vi "reconCluster.vi"(7 "Array 6":bool[](array[boolean]), 8 "Variable header":string[](array[string]), 9 "Alias":string[](array[string]), 10 "Data in":string[][](array[string]), 11 "variant in":variant) -> (1 "time":u32, 3 "variant out":variant)   [LabVIEW 2013]
uses:
  IMAQ Image.ctl
  NI_Vision_Development_Module.lvlib
panel:
  out "Img str lengths":i32[](array[numeric])
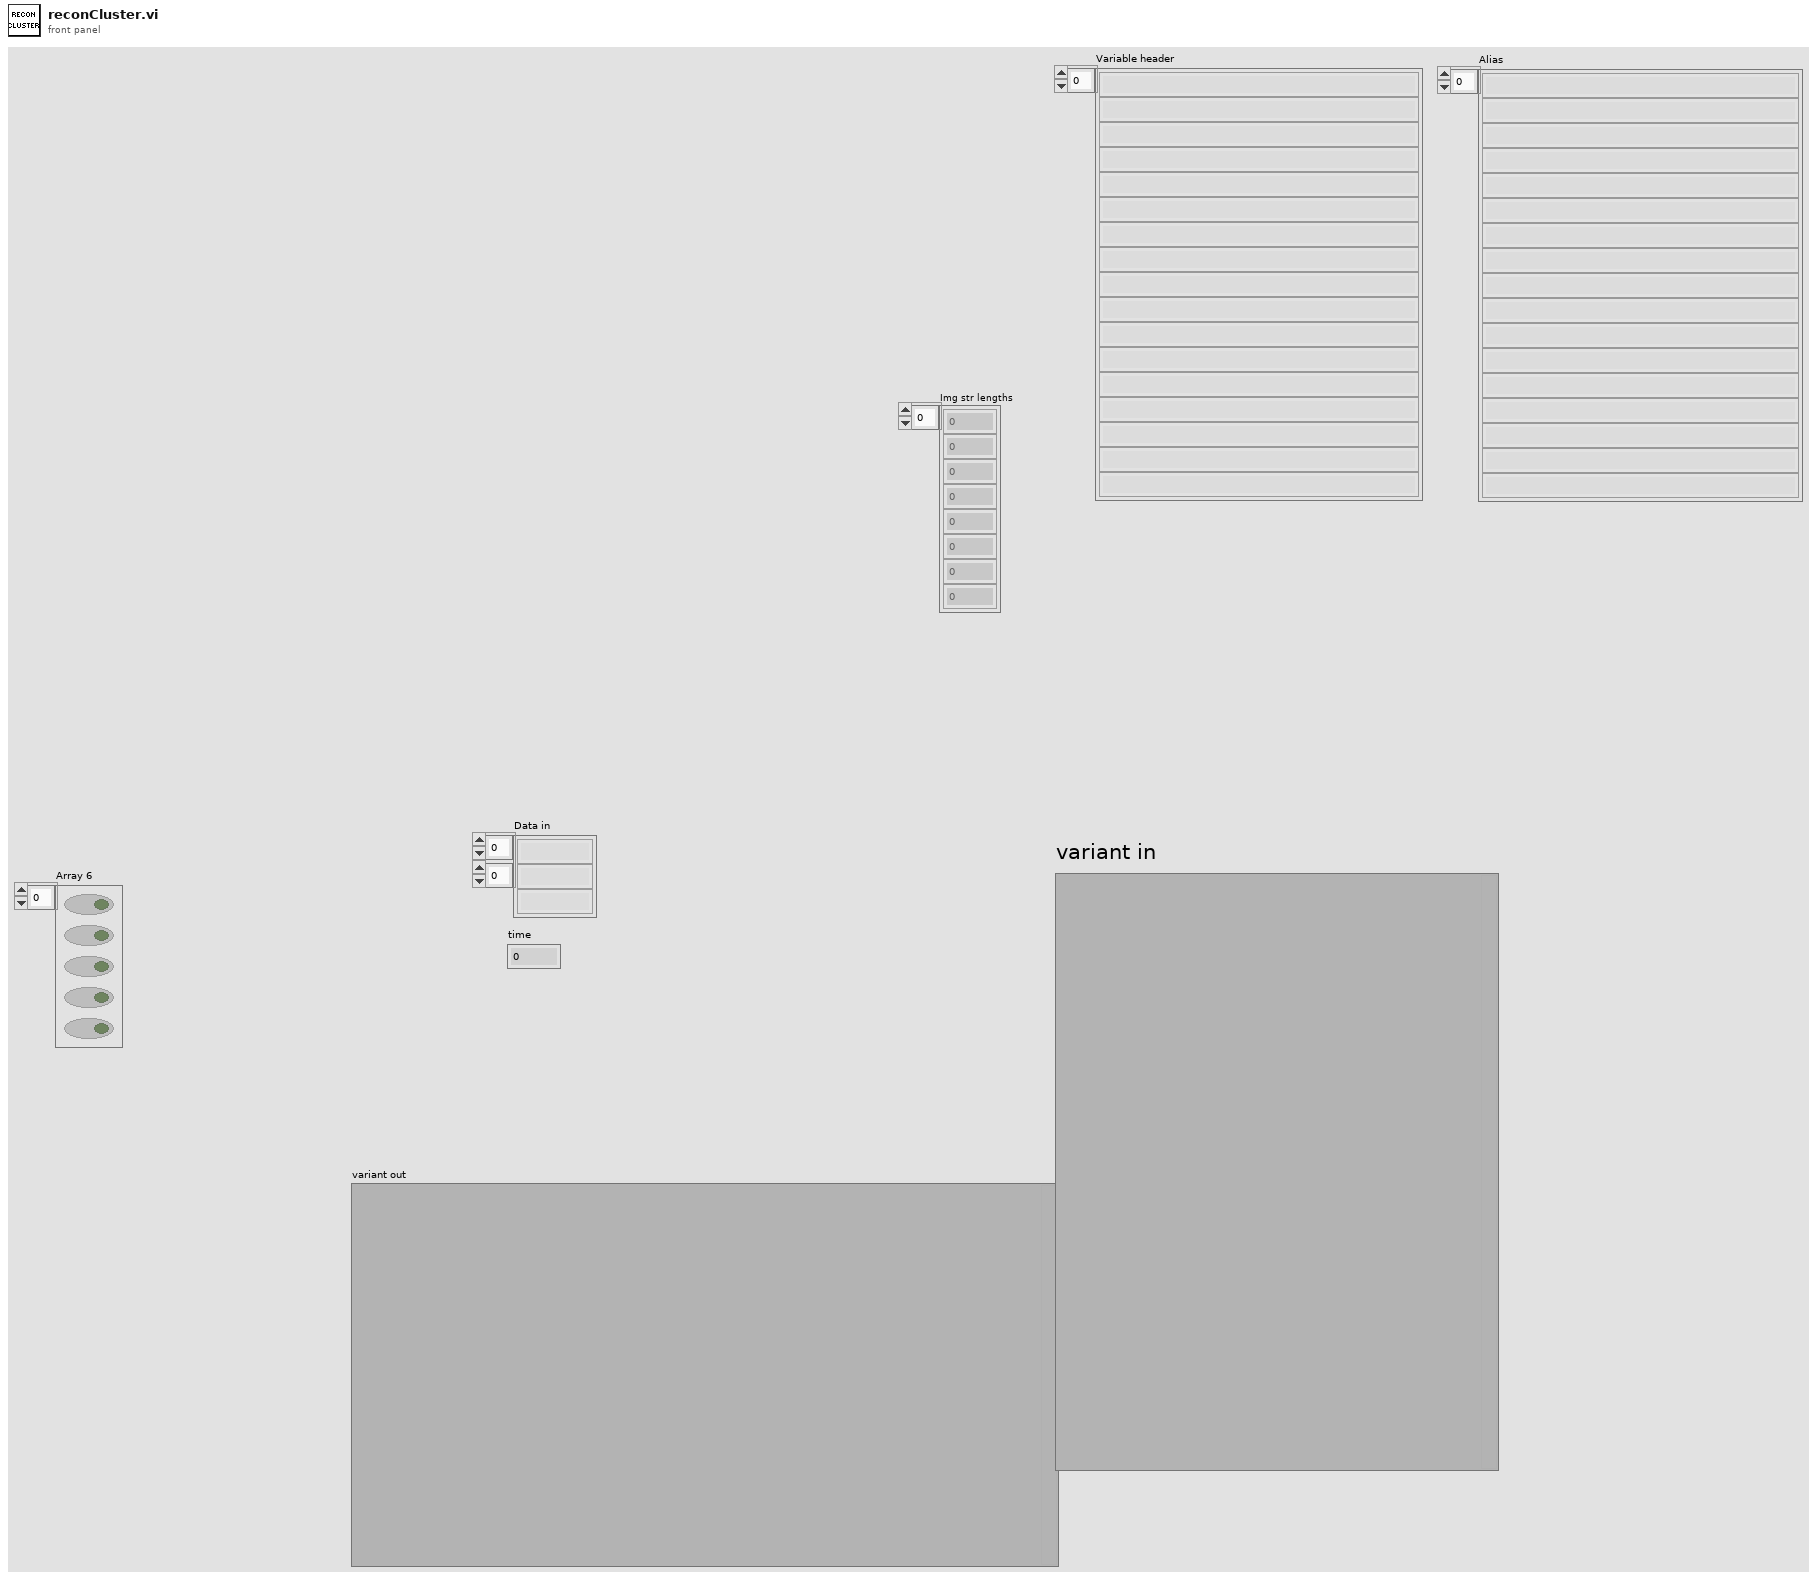
[diagram p1: front panel]
types:
  T1 = typedef "IMAQ Image.ctl" = refnum<image>
  T2 = typedef "Type Descriptor Enumeration__ogtk.ctl" = enum8{"<Null>", "I8", "I16", "I32", "I64", "U8", "U16", "U32", "U64", "SGL", "DBL", "EXT", "CSG", "CDB", "CXT", "0x0F", "0x10", "0x11", "0x12", "0x13", "0x14", "Enum U8", "Enum U16", "Enum U32", "Enum U64", "SGL PQ", "DBL PQ", "EXT PQ", "CSG PQ", "CDB PQ", "CXT PQ", "0x1F", "0x20", "Boolean", "0x22", "0x23", "0x24", "0x25", "0x26", "0x27", "0x28", "0x29", "0x2A", "0x2B", "0x2C", "0x2D", "0x2E", "0x2F", "String", "0x31", "Path", "Pict", "0x34", "0x35", "0x36", "DAQ", "0x38", "0x39", "0x3A", "0x3B", "0x3C", "0x3D", "0x3E", "0x3F", "Array", "0x41", "0x42", "0x43", "0x44", "0x45", "0x46", "0x47", "0x48", "0x49", "0x4A", "0x4B", "0x4C", "0x4D", "0x4E", "0x4F", "Cluster", "0x51", "0x52", "Variant", "Waveform", "0x55", "0x56", "0x57", "0x58", "0x59", "0x5A", "0x5B", "0x5C", "0x5D", "0x5E", "0x5F", "0x60", "0x61", "0x62", "0x63", "0x64", "0x65", "0x66", "0x67", "0x68", "0x69", "0x6A", "0x6B", "0x6C", "0x6D", "0x6E", "0x6F", "Refnum"}
  T3 = typedef "Image Type" = u32
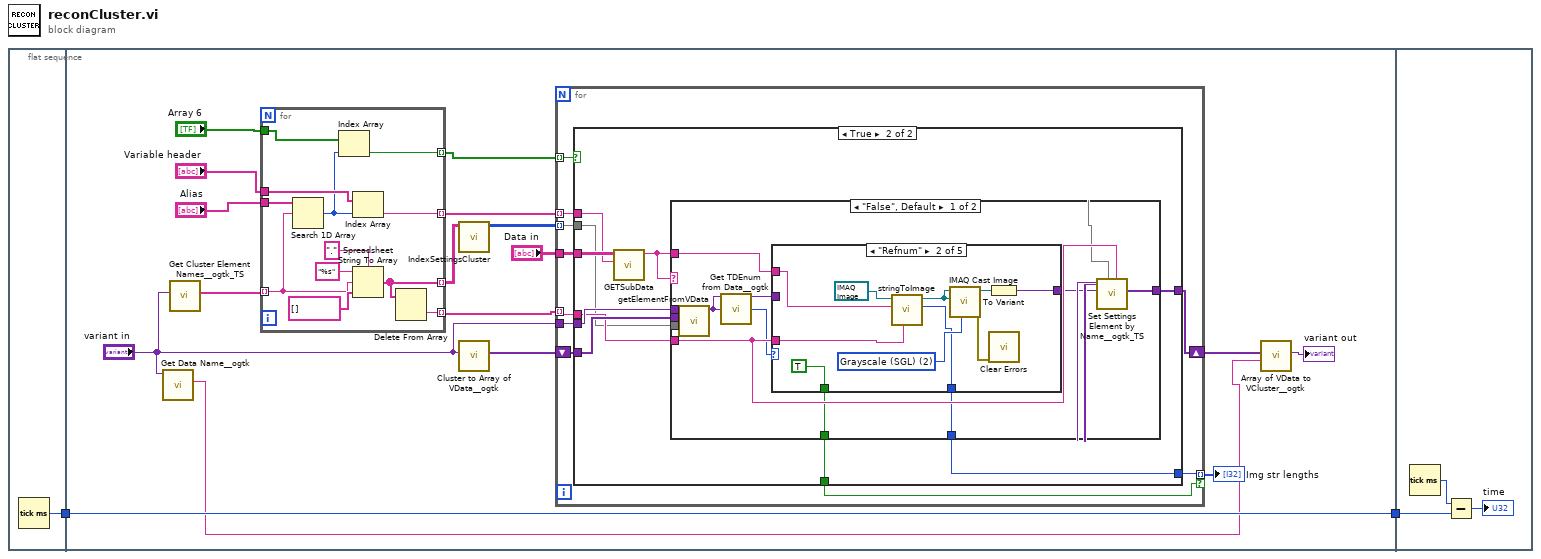
[diagram p0: block diagram]
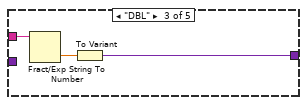
[diagram p4: hidden frame]
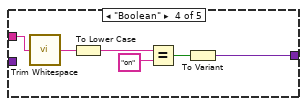
[diagram p5: hidden frame]
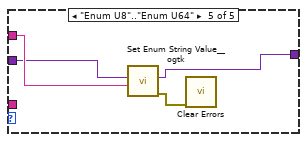
[diagram p6: hidden frame]
diagram:
  n1 = flat-sequence {
    tunnel: [w3] -> w2
    tunnel: w2 -> [w13]
    tunnel: [w13] -> w1
    tunnel: w1 -> [w90]
    frame #0 {
      n2 = Tick Count (ms)() -> (millisecond timer value=w3:u32)
    }
    frame #1 {
      n3 = call "Get Data Name__ogtk.vi"("Data"="variant in") -> ("Data Name"=w7:string)  [unwired: 8 in, 2 out]
      n4 = call "Get Cluster Element Names__ogtk_TS.vi"("Variant"="variant in") -> ("Names (Array)"=w19:string[])  [unwired: 9 in, 1 out]
      n5 = for {
        tunnel: w19 -> [w82] mode=indexing
        tunnel: [w85] -> w20 mode=indexing
        tunnel: [w84] -> w16 mode=indexing
        tunnel: "Alias" -> [w83]
        tunnel: "Variable header" -> [w81]
        tunnel: [w80] -> w9 mode=indexing
        tunnel: "Array 6" -> [w79]
        tunnel: [w77] -> w5 mode=indexing
        n6 = Search 1D Array(1D array=w83, element=w82) -> (index of element=w78:i32)  [unwired: 1 in]
        n7 = Index Array(array=w79, index=w78) -> (element=w77:bool)
        n8 = Index Array(array=w81, index=w78) -> (element=w80:string)
        n9 = Spreadsheet String To Array(delimiter (Tab)=".", format string="%s", spreadsheet string=w82, array type (2D Dbl)=string[] []) -> (array=w85:string[])
        n10 = Delete From Array(array=w85) -> (deleted portion=w84:string)  [unwired: 2 in, 1 out]
      }
      n11 = call "IndexSettingsCluster.vi"("Names Array"=w20) -> ("index Array"=w17:i32[][])  [unwired: 10 in]
      n12 = call "Cluster to Array of VData__ogtk.vi"("Cluster"="variant in") -> ("Array of VData"=w18:variant[])  [unwired: 9 in, 1 out]
      n13 = for {
        shift-right: [w30] -> w15
        shift-left: w18 -> [w28]
        tunnel: w17 -> [w27] mode=indexing
        tunnel: "variant in" -> [w29]
        tunnel: w16 -> [w24] mode=indexing
        tunnel: "Data in" -> [w26]
        tunnel: w9 -> [w25] mode=indexing
        tunnel: w5 -> [w23] mode=indexing
        tunnel: [w22] -> w4 mode=indexing if=w21
        n14 = case shown="True" w23 {
          tunnel: [w31 w41] -> w30
          tunnel: w29 -> [_ w40]
          tunnel: w28 -> [w31 w39]
          tunnel: w27 -> [_ w35]
          tunnel: w26 -> [_ w38]
          tunnel: w25 -> [_ w37]
          tunnel: w24 -> [_ w36]
          tunnel: [_ w33] -> w21
          tunnel: [_ w32] -> w22
          frame False {
          }
          frame True {
            n15 = call "GETSubData.vi"("Variable Header"=w37, "Data out"=w38) -> ("delimiter (Tab)"=w34:string)  [unwired: 9 in]
            n16 = case shown="\"False\", Default" w34 {
              tunnel: [w52 _] -> w41
              tunnel: w40 -> [w51 _]
              tunnel: w39 -> [w50 _]
              tunnel: w34 -> [w49 _]
              tunnel: w36 -> [w48 _]
              tunnel: w35 -> [w44 _]
              tunnel: [w43 _] -> w33
              tunnel: [w42 _] -> w32
              frame "False", Default {
                n17 = call "getElementFromVData.vi"("index Array 2"=w44, "Settings VData"=w50, "Cluster in"=w51) -> ("element out"=w45:variant)  [unwired: 6 in, 2 out]
                n18 = call "Get TDEnum from Data__ogtk.vi"("Data"=w45) -> ("Type Descriptor Enumeration"=w47:T2)  [unwired: 4 in]
                n19 = case shown="\"Refnum\"" w47 {
                  tunnel: w49 -> [_ w63 w66 w72 w76]
                  tunnel: w48 -> [_ w57 _ _ _]
                  tunnel: [w53 w58 w64 w67 w74] -> w46
                  tunnel: w45 -> [w53 _ _ _ w75]
                  tunnel: [_ TRUE ("element") _ _ _] -> w43
                  tunnel: [_ w54 _ _ _] -> w42
                  frame "<Null>", Default {
                  }
                  frame "Refnum" {
                    w61 = T3 2 items=["Grayscale (U8)", "Grayscale (I16)", "Grayscale (SGL)", "Complex (CSG)", "RGB (U32)", "HSL (U32)", "RGB (U64)", "Grayscale (U16)"] ("Image Type")
                    n20 = call "stringToImage.vi"("label text (image name)"=w57, "data in"=w63, "Refnum in"=T1 refnum ("Image")) -> ("length"=w54:i32, "Refnum out"=w62:T1)  [unwired: 5 in, 2 out]
                    n21 = call "IMAQ Cast Image"("Image Type"=w61, "Image Dst"=w62, "Image Src"=w62) -> ("error out"=w56:errorcluster, "Image Dst Out"=w59:T1)  [unwired: 7 in]
                    n22 = To Variant(anything=w59) -> (Variant=w58:variant)
                    n23 = call "Clear Errors.vi"("error in (no error)"=w56) -> ()  [unwired: 6 in, 1 out]
                  }
                  frame "DBL" {
                    n24 = Fract/Exp String To Number(string=w66) -> (number=w65:dbl)  [unwired: 3 in, 1 out]
                    n25 = To Variant(anything=w65) -> (Variant=w64:variant)
                  }
                  frame "Boolean" {
                    n26 = call "Trim Whitespace.vi"("string"=w72) -> ("trimmed string"=w71:string)  [unwired: 1 in]
                    n27 = To Lower Case(string=w71) -> (all lower case string=w70:string)
                    n28 = Equal?(x=w70, y="on" ("x")) -> (x = y?=w68:bool)
                    n29 = To Variant(anything=w68) -> (Variant=w67:variant)
                  }
                  frame "Enum U8".."Enum U64" {
                    n30 = call "Set Enum String Value__ogtk.vi"("String Value"=w76, "Default Enum Value"=w75) -> ("error out"=w73:errorcluster, "Enum"=w74:variant)  [unwired: 8 in]
                    n31 = call "Clear Errors.vi"("error in (no error)"=w73) -> ()  [unwired: 6 in, 1 out]
                  }
                }
                n32 = call "Set Settings Element by Name__ogtk_TS.vi"("element Name"=w48, "index Array"=w44, "Settings VData"=w50, "New Element Value"=w46, "Cluster"=w51) -> ("Settings VData out"=w52:variant[])  [unwired: 5 in, 1 out]
              }
              frame "n/a" {
              }
            }
          }
        }
      }
      "Img str lengths" <- w4
      n33 = call "Array of VData to VCluster__ogtk.vi"("Cluster Name"=w7, "Array"=w15) -> ("VCluster"=→"variant out":variant)  [unwired: 8 in, 1 out]
    }
    frame #2 {
      n34 = Tick Count (ms)() -> (millisecond timer value=w91:u32)
      n35 = Subtract(x=w91, y=w90) -> (x-y=→"time":u32)
    }
  }
